vi "get_time_and_rate.vi"(8 "error in (no error)":errorcluster, 9 "Status":T1, 10 "Threads (32)":i32=32, 11 "ID":i32) -> (0 "error out":errorcluster, 1 "Scan result":cluster{"Time (DBL)":dbl[], "Video ID":i32[]}, 2 "ID rate (per second)":dbl, 3 "ID timestamp":timestamp)   [LabVIEW 2023]
uses:
  <vilib>/Analysis/6fits.llb/Curve Fitting Criteria.ctl
  <vilib>/gmath/statdist.llb/st_Percentiles (scalar).vi
  <vilib>/httpClient/LabVIEWHTTPClient.lvlib
  <vilib>/Analysis/NI_AALPro.lvlib
  <vilib>/gmath/NI_Gmath.lvlib
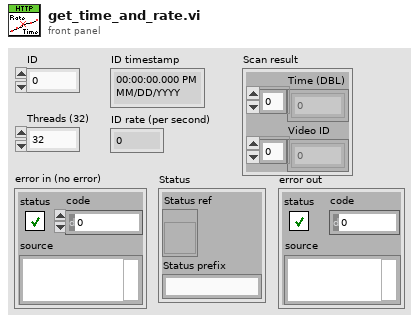
[diagram p1: front panel]
types:
  T1 = cluster{"Status ref":refnum<vi>, "Status prefix":string}
  T2 = typedef "NI_AALPro.lvlib/Curve Fitting Criteria.ctl" = u16
  T3 = typedef "LabVIEWHTTPClient.lvlib/ClientHandle.ctl" = refnum<k1>
  T4 = cluster{"Title":string, "Channel":string, "Duration (s)":i32, "Is streaming":bool, "Timestamp":timestamp}
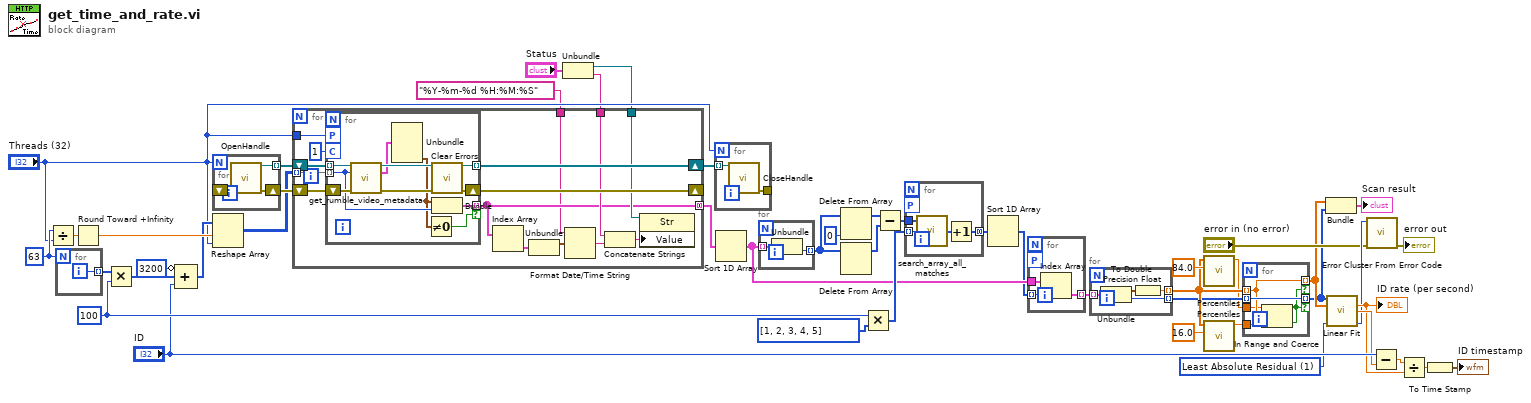
[diagram p0: block diagram]
diagram:
  w19 = T2 1 items=["Least Square", "Least Absolute Residual", "Bisquare"] ("method")
  w43 = 63
  w26 = 100
  n1 = Divide(x=w43, y="Threads (32)") -> (x/y=w45:dbl)
  n2 = for {
    N: w43 -> [_]
    tunnel: [w49] -> w47 mode=indexing
    i -> [w49]
  }
  n3 = Round Toward +Infinity(x=w45) -> (ceil(x): smallest int >= x=w44:dbl)
  n4 = Multiply(x=w47, y=w26) -> (x*y=w46:i32[])
  n5 = Compound Arithmetic op=ADD(invert 3200 ("y"), w46, "ID") -> (w42:i32[])
  n6 = for {
    N: "Threads (32)" -> [_]
    tunnel: [w52] -> w41 mode=indexing
    shift-right: [w51] -> w40
    shift-left: _ -> [w50]
    n7 = call <vilib>:"OpenHandle.vi"("error in (no error)"=w50) -> ("client handle out"=w52:T3, "error out"=w51:errorcluster)  [unwired: 13 in]
  }
  n8 = Reshape Array(w42, w44, "Threads (32)") -> (w28:i32[][])
  n9 = Unbundle("Status") -> ("Status ref"=w2:refnum<vi>, "Status prefix"=w3:string)
  n10 = for {
    tunnel: "Threads (32)" -> [w64]
    shift-right: [w65] -> _
    shift-left: w40 -> [w66]
    shift-right: [w63] -> w39
    shift-left: w41 -> [w67]
    tunnel: w28 -> [w61] mode=indexing
    tunnel: [w57] -> w30 mode=concatenating
    tunnel: w3 -> [w60]
    tunnel: w2 -> [w59]
    tunnel: "%Y-%m-%d %H:%M:%S" ("time format string (%c)") -> [w54]
    n11 = for {
      shift-right: [w70] -> w65
      shift-left: w66 -> [w76]
      workers-P: w64 -> [_]
      tunnel: w61 -> [w71] mode=indexing
      tunnel: w67 -> [w77] mode=indexing
      tunnel: [w75] -> w63 mode=indexing
      chunk-C: 1 -> [_]
      tunnel: [w73] -> w57 mode=indexing if=w68
      n12 = call "get_rumble_video_metadata.vi"("HTTP client handle"=w77, "Video ID"=w71, "error in (no error)"=w76) -> ("client handle out"=w75:T3, "Video metadata"=w74:T4, "error out"=w72:errorcluster)  [unwired: 8 in, 2 out]
      n13 = Unbundle(w74) -> ("Timestamp"=w69:timestamp)  [unwired: 4 out]
      n14 = Not Equal To 0?(x=w69) -> (x != 0?=w68:bool)
      n15 = call <vilib>:"Clear Errors.vi"("error in (no error)"=w72) -> ("error out"=w70:errorcluster)  [unwired: 5 in, 1 out]
      n16 = Bundle("Timestamp"=w69, w71) -> (w73:cluster{"Timestamp":timestamp, i32})  [unwired: 1 in]
    }
    n17 = Index Array(array=w57) -> (element=w56:cluster{"Timestamp":timestamp, i32})  [unwired: 1 in]
    n18 = Unbundle(w56) -> ("Timestamp"=w55:timestamp)  [unwired: 1 out]
    n19 = Format Date/Time String(time format string (%c)=w54, seconds (now)=w55) -> (date/time string=w53:string)  [unwired: 1 in]
    n20 = Concatenate Strings(w60, w53) -> (w58:string)
    n21 = property class="Str"(reference=w59, "Value"=w58) -> ()  [unwired: 1 in, 2 out]
  }
  n22 = for {
    N: "Threads (32)" -> [_]
    tunnel: w39 -> [w79] mode=indexing
    tunnel: [w78] -> _
    n23 = call <vilib>:"CloseHandle.vi"("client handle"=w79) -> ("error out"=w78:errorcluster)  [unwired: 14 in]
  }
  n24 = Sort 1D Array(array=w30) -> (sorted array=w31:cluster{"Timestamp":timestamp, i32}[])
  n25 = for {
    tunnel: w31 -> [w81] mode=indexing
    tunnel: [w80] -> w38 mode=indexing
    n26 = Unbundle(w81) -> (w80:i32)  [unwired: 1 out]
  }
  n27 = Delete From Array(array=w38, index=0) -> (array with subset deleted=w36:i32[])  [unwired: 1 in, 1 out]
  n28 = Delete From Array(array=w38) -> (array with subset deleted=w35:i32[])  [unwired: 2 in, 1 out]
  n29 = Multiply(x=w26, y=i32[] [1, 2, 3, 4, 5]) -> (x*y=w32:i32[])
  n30 = Subtract(x=w36, y=w35) -> (x-y=w34:i32[])
  n31 = for {
    tunnel: w34 -> [w84]
    workers-P: _ -> [_]
    tunnel: w32 -> [w83] mode=indexing
    tunnel: [w85] -> w29 mode=concatenating
    n32 = call "search_array_all_matches.vi"("Array"=w84, "Element Data"=w83) -> ("Indices of Elements"=w82:i32[])  [unwired: 7 in]
    n33 = Increment(x=w82) -> (x+1=w85:i32[])
  }
  n34 = Sort 1D Array(array=w29) -> (sorted array=w14:i32[])
  n35 = for {
    tunnel: w14 -> [w88] mode=indexing
    tunnel: w31 -> [w87]
    tunnel: [w86] -> w13 mode=indexing
    workers-P: _ -> [_]
    n36 = Index Array(array=w87, index=w88) -> (element=w86:cluster{"Timestamp":timestamp, i32})
  }
  n37 = for {
    tunnel: w13 -> [w92] mode=indexing
    tunnel: [w91] -> w9 mode=indexing
    tunnel: [w90] -> w10 mode=indexing
    n38 = Unbundle(w92) -> ("Timestamp"=w89:timestamp, w91:i32)
    n39 = To Double Precision Float(number=w89) -> (double precision float=w90:dbl)
  }
  n40 = call-poly <vilib>:"Percentiles.vi"("p"=84.0, "x array"=w10) -> ("percentile"=w8:dbl)  [unwired: 8 in, 1 out]
  n41 = call-poly <vilib>:"Percentiles.vi"("p"=16.0, "x array"=w10) -> ("percentile"=w7:dbl)  [unwired: 8 in, 1 out]
  n42 = for {
    tunnel: [w97] -> w5 mode=indexing if=w93
    tunnel: w10 -> [w96] mode=indexing
    tunnel: w9 -> [w97] mode=indexing
    tunnel: [w96] -> w6 mode=indexing if=w93
    tunnel: w8 -> [w95]
    tunnel: w7 -> [w94]
    n43 = In Range and Coerce(upper limit=w95, x=w96, lower limit=w94) -> (In Range?=w93:bool)  [unwired: 1 out]
  }
  n44 = Bundle(w6, w5) -> (→"Scan result":cluster{dbl[], i32[]})  [unwired: 1 in]
  n45 = call <vilib>:"Linear Fit.vi"("Y"=w5, "X"=w6, "method"=w19) -> ("slope"=w21:dbl, "intercept"=w24:dbl, "error"=w18:i32)  [unwired: 8 in, 2 out]
  "ID rate (per second)" <- w21
  n46 = call <vilib>:"Error Cluster From Error Code.vi"("error in (no error)"="error in (no error)", "error code (0)"=w18) -> ("error out"=→"error out":errorcluster)  [unwired: 7 in]
  n47 = Subtract(x="ID", y=w24) -> (x-y=w23:dbl)
  n48 = Divide(x=w23, y=w21) -> (x/y=w20:dbl)
  n49 = To Time Stamp(1:w20) -> (0:→"ID timestamp":timestamp)
